vi "Delete Elements from 1D Array (I8)__ogtk.vi"(9 "indices":i32[](array[numeric]), 11 "array":i8[](array[numeric])) -> (1 "deleted elements":i8[](array[numeric]), 3 "array w/ subset deleted":i8[](array[numeric]))   [LabVIEW 2012]
doc: "This polymorphic VI deletes elements from a 1D or 2D <B>array</B> at the corresponding <B>indices</B>, returning <B>array w/ subset deleted</B> and <B>deleted elements</B>. For 2D arrays, wire the <B>delete (rows or columns)</B> input to specify whether to delete rows or columns."
uses:
  <userlib>/_OpenG.lib/array/array.llb/Sort 1D Array (I32)__ogtk.vi
  <userlib>/_OpenG.lib/array/array.llb/Reorder 1D Array2 (I8)__ogtk.vi
panel:
  # "Delete Elements from Array.vi\n\nThis polymorphic VI deletes elements from a 1D or 2D array at the corresponding indices\n\nPlease visit http://www.OpenG.org to learn about the\nOpen Source LabVIEW software movement.\n\nNOTICE -- YOU MUST LEAVE THIS NOTICE IN PLACE.  PER THE TERMS OF THE LICENSE BELOW, YOU MAY SUBLICENSE THIS SOFTWARE \nIN ANY WAY THAT DOES NOT CONFLICT WITH THIS LICENSE.\n\n### BSD License (http://www.opensource.org/licenses/bsd-license.php) Begin ###\n \nCopyright (c) 2007, JKI <info@jameskring.com> (Author: Jim Kring <jim.kring@jameskring.com>)\n\nAll rights reserved.\n\nRedistribution and use in source and binary forms, with or without modification, are permitted provided that the following conditions are met:\n\n    * Redistributions of source code must retain the above copyright notice, this list of conditions and the following disclaimer.\n    * Redistributions in binary form must reproduce the above copyright notice, this list of conditions and the following disclaimer in the \n       documentation and/or other materials provided with the distribution.\n    * Neither the name of SciWare, James Kring, Inc., nor the names of its contributors may be used to endorse or promote products derived \n       from this software without specific prior written permission.\n\nTHIS SOFTWARE IS PROVIDED BY THE COPYRIGHT HOLDERS AND CONTRIBUTORS \"AS IS\" AND ANY EXPRESS OR IMPLIED WARRANTIES, \nINCLUDING, BUT NOT LIMITED TO, THE IMPLIED WARRANTIES OF MERCHANTABILITY AND FITNESS FOR A PARTICULAR PURPOSE ARE \nDISCLAIMED. IN NO EVENT SHALL THE COPYRIGHT OWNER OR CONTRIBUTORS BE LIABLE FOR ANY DIRECT, INDIRECT, INCIDENTAL,\n SPECIAL, EXEMPLARY, OR CONSEQUENTIAL DAMAGES (INCLUDING, BUT NOT LIMITED TO, PROCUREMENT OF SUBSTITUTE GOODS OR \nSERVICES; LOSS OF USE, DATA, OR PROFITS; OR BUSINESS INTERRUPTION) HOWEVER CAUSED AND ON ANY THEORY OF LIABILITY, \nWHETHER IN CONTRACT, STRICT LIABILITY, OR TORT (INCLUDING NEGLIGENCE OR OTHERWISE) ARISING IN ANY WAY OUT OF THE USE \nOF THIS SOFTWARE, EVEN IF ADVISED OF THE POSSIBILITY OF SUCH DAMAGE.\n\n### BSD License End ###"
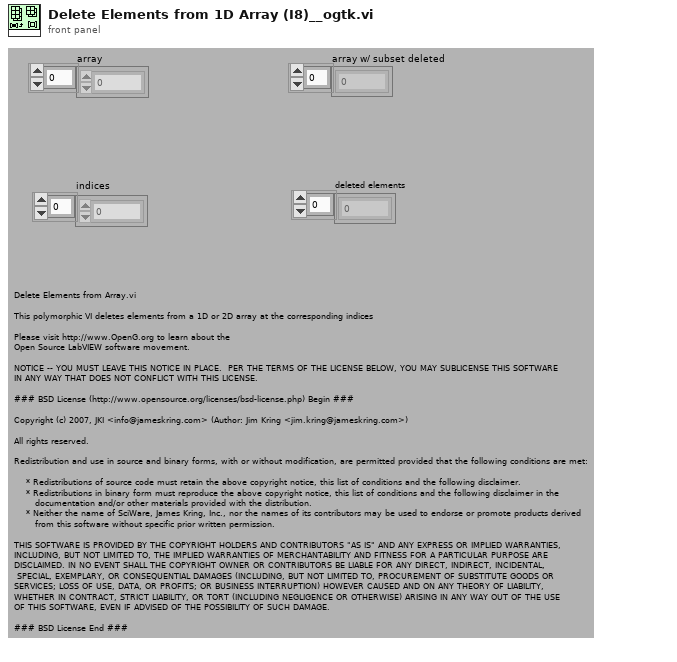
[diagram p1: front panel]
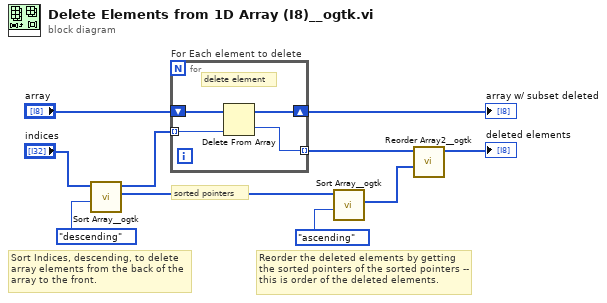
[diagram p0: block diagram]
diagram:
  # "Reorder the deleted elements by getting the sorted pointers of the sorted pointers -- this is order of the deleted elements."
  # "Sort Indices, descending, to delete array elements from the back of the array to the front."
  # "sorted pointers"
  n1 = call-poly <userlib>:"Sort Array__ogtk.vi"("Order"=enum16{"ascending", "descending"}."descending", "Array in"="indices") -> ("Sorted Pointers"=w4:i32[], "Sorted Array out"=w6:i32[])  [unwired: 8 in]
  n2 = for "For Each element to delete" {
    tunnel: w6 -> [w14] mode=indexing
    shift-right: [w13] -> w9
    shift-left: "array" -> [w12]
    tunnel: [w11] -> w3 mode=indexing
    # "delete element"
    n3 = Delete From Array(array=w12, index=w14) -> (deleted portion=w11:i8, array with subset deleted=w13:i8[])  [unwired: 1 in]
  }
  "array w/ subset deleted" <- w9
  n4 = call-poly <userlib>:"Sort Array__ogtk.vi"("Order"=enum16{"ascending", "descending"}."ascending", "Array in"=w4) -> ("Sorted Pointers"=w1:i32[])  [unwired: 8 in, 1 out]
  n5 = call-poly <userlib>:"Reorder Array2__ogtk.vi"("indices"=w1, "array"=w3) -> ("reordered array"=→"deleted elements":i8[])  [unwired: 9 in]
